vi "GlobalPhoneNumber.vi"() -> ()   [LabVIEW 2017]
panel:
  out "Phone number":string
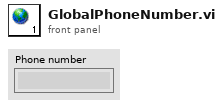
[diagram p1: front panel]
diagram:
